vi "_32_Sample_qsns_9[8].vi"() -> ()   [LabVIEW 2020]
panel:
  out "element":i32
  out "Waveform Graph":i32[](graph)
  out "Boolean":bool
  out "Numeric":i32
  out "Numeric 2":i32
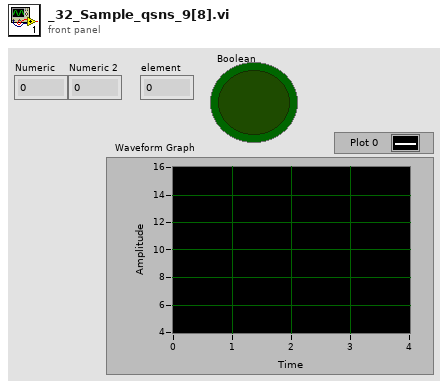
[diagram p1: front panel]
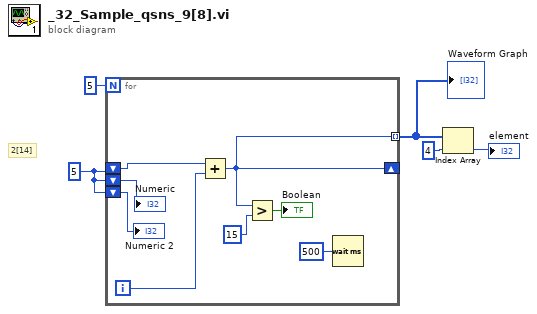
[diagram p0: block diagram]
diagram:
  w4 = 5
  # "2[14]"
  n1 = for {
    N: 5 -> [_]
    shift-right: [w7] -> _
    shift-left: w4 -> [w10]
    shift-left: w4 -> [w9]
    shift-left: w4 -> [w8]
    tunnel: [w7] -> w2 mode=indexing
    i -> [w11]
    n2 = Add(x=w10, y=w11) -> (x+y=w7:i32)
    n3 = Greater?(x=w7, y=15) -> (0:→"Boolean":bool)
    n4 = Wait (ms)(milliseconds to wait=u32 500) -> ()  [unwired: 1 out]
    "Numeric" <- w9
    "Numeric 2" <- w8
  }
  "Waveform Graph" <- w2
  n5 = Index Array "Index Array"(array=w2, index=4) -> (element=→"element":i32)
